vi "Controller Write PS Setpoints.vi"(0 "PS Setpoint Variables":refnum<k21>[](array[refnum]), 2 "PS Setpoints":dbl[](array[numeric]), 3 "error in (no error)":errorcluster) -> (10 "error out":errorcluster)   [LabVIEW 2011, in "Controller VIs.lvlib"]
doc: "Writes PS Setpoints variables to the Actuation chassis."
uses:
  Controller VIs.lvlib
  Simulated Beam VIs/Simulated PS Current.vi
  Simulated Beam VIs.lvlib
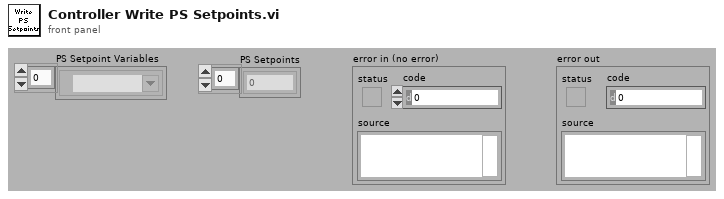
[diagram p1: front panel]
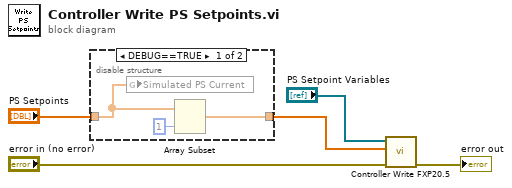
[diagram p0: block diagram]
diagram:
  n1 = disable-structure shown="DEBUG==TRUE" {
    disable-tunnel: "PS Setpoints" -> [w8 w9]
    disable-tunnel: [w6 w9] -> w1
    frame condition #0 {
      n2 = global write "Simulated PS Current.vi" "Simulated PS Current"(w8) -> ()
      n3 = Array Subset(array=w8, length=1) -> (w6:dbl[])  [unwired: 1 in]
    }
    frame condition #1 (active) {
    }
  }
  n4 = call "Controller Write FXP20.5.vi"("Error In"="error in (no error)", "Values"=w1, "Variables"="PS Setpoint Variables") -> ("Error Out"=→"error out":errorcluster)  [unwired: 8 in]
